vi "get list with seq.vi"(9 "charge state":string, 10 "wheelnumber":string, 11 "runletter":string) -> (3 "Array":string[][](array[string]))   [LabVIEW 2016]
uses:
  <vilib>/addons/database/Connection.llb/DB Tools Open Connec (String).vi
  <vilib>/addons/database/Connection.llb/Conn Execute.vi
  <vilib>/addons/database/Recordset.llb/Rec Fetch Recordset Data (R).vi
  <vilib>/addons/database/Recordset.llb/Rec Destroy - Connection.vi
  <vilib>/addons/database/NI_Database_API.lvlib
  <vilib>/Analysis/NI_AALBase.lvlib
panel:
  out "error out":errorcluster
  out "recordset data":variant[][](array[variant])
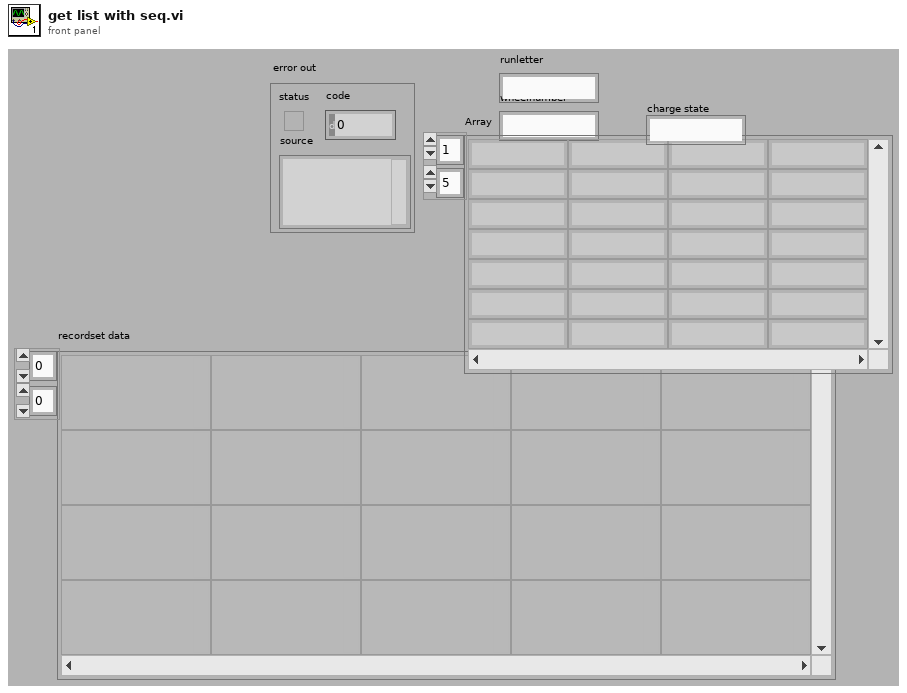
[diagram p1: front panel]
types:
  T1 = typedef "NI_Database_API.lvlib/Conn ObjectReference.ctl" = refnum<k1>
  T2 = typedef "NI_Database_API.lvlib/Rec ObjectReference.ctl" = refnum<k1>
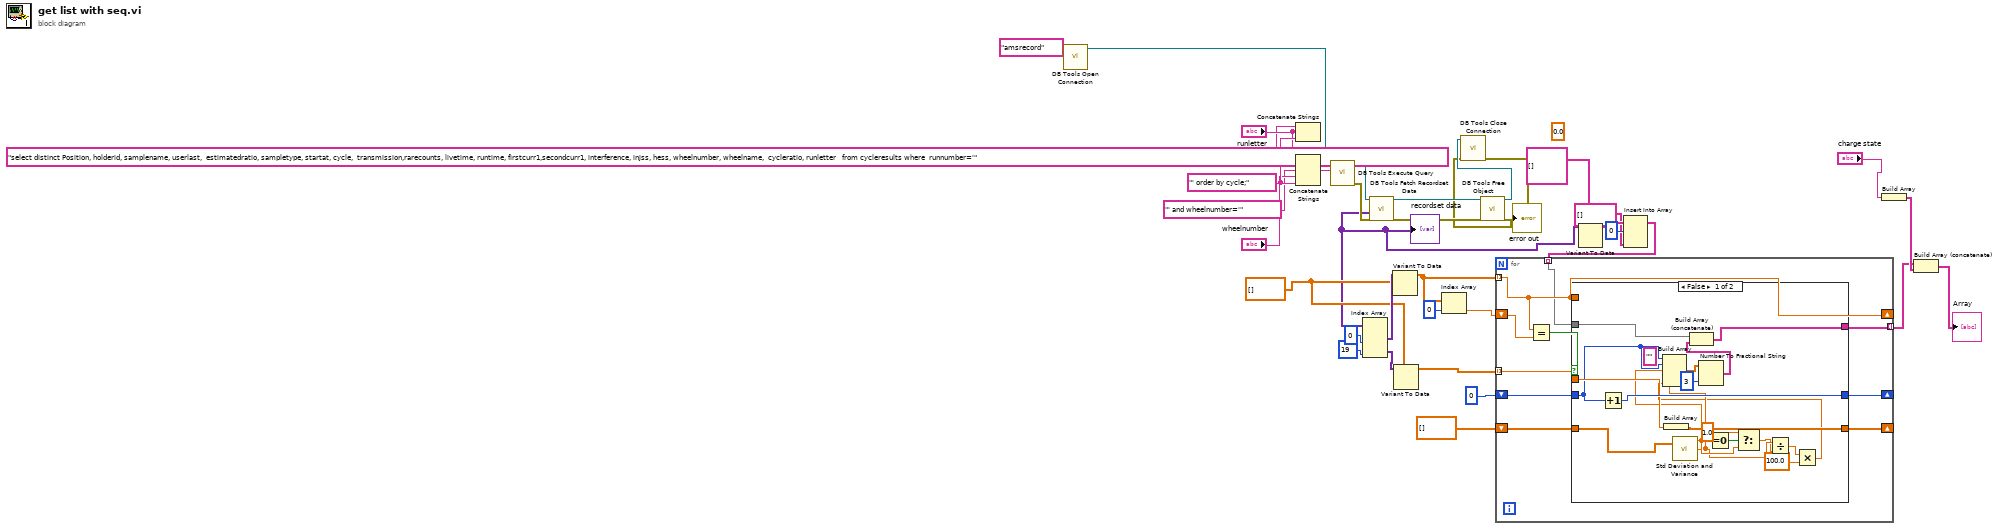
[diagram p0: block diagram]
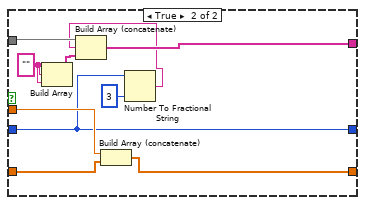
[diagram p2: hidden frame]
diagram:
  (unwired) 0.0
  w21 = dbl[] []
  w34 = "' order by cycle;" ("SQL query get data name")
  w32 = "select distinct Position, holderid, samplename, userlast,  estimatedratio, sampletype, startat, cycle,  transmission,rarecounts, livetime, runtime, firstcurr1,secondcurr1, interference, injss, hess, wheelnumber, wheelname,  cycleratio, runletter   from cycleresults where  runnumber='" ("SQL query get data name")
  n1 = call-poly <vilib>:"DB Tools Open Connection.vi"("connection information"="amsrecord") -> ("connection reference"=w27:T1)  [unwired: 7 in, 1 out]
  n2 = Concatenate Strings(w32, "runletter", w34) -> ()  [unwired: 1 out]
  n3 = Concatenate Strings(w32, "runletter", "' and wheelnumber='" ("SQL query get data name"), "wheelnumber", w34) -> (w35:string)
  n4 = call-poly <vilib>:"DB Tools Execute Query.vi"("SQL query"=w35, "connection reference"=w27) -> ("error out"=w28:errorcluster, "recordset reference"=w29:T2)  [unwired: 6 in]
  n5 = call-poly <vilib>:"DB Tools Fetch Recordset Data.vi"("error in (no error)"=w28, "recordset reference"=w29) -> ("error out"=w25:errorcluster, "recordset data"=w13:variant[][], "recordset reference out"=w26:T2)  [unwired: 3 in]
  "recordset data" <- w13
  n6 = Index Array(array=w13, index (col) #1=0 ("index (row)"), index (col) #2=19 ("disabled index (col)")) -> (element #1=w22:variant[], element #2=w20:variant[])  [unwired: 2 in]
  n7 = Variant To Data(type=w21, Variant=w22) -> (data=w17:dbl[])  [unwired: 1 in, 1 out]
  n8 = Variant To Data(type=w21, Variant=w20) -> (data=w19:dbl[])  [unwired: 1 in, 1 out]
  n9 = Index Array(array=w17, index=0) -> (element=w15:dbl)
  n10 = call-poly <vilib>:"DB Tools Free Object.vi"("error in (no error)"=w25, "recordset reference"=w26) -> ("error out"=w1:errorcluster, "connection reference"=w3:T1)  [unwired: 8 in]
  n11 = call <vilib>:"DB Tools Close Connection.vi"("error in (no error)"=w1, "connection reference"=w3) -> ("error out"=→"error out":errorcluster)  [unwired: 5 in]
  n12 = Variant To Data(type=string[][] [], Variant=w13) -> (data=w11:string[][])  [unwired: 1 in, 1 out]
  n13 = Insert Into Array(array=w11, index (row)=0, new element=string[] [] ("new element/subarray")) -> (w8:string[][])  [unwired: 1 in]
  n14 = for {
    tunnel: w19 -> [w42] mode=indexing
    tunnel: w17 -> [w44] mode=indexing
    shift-right: [w39] -> _
    shift-left: 0 ("index (row)") -> [w46]
    shift-right: [w44] -> _
    shift-left: w15 -> [w45]
    shift-right: [w40] -> _
    shift-left: dbl[] [] -> [w41]
    tunnel: w8 -> [w38] mode=indexing
    tunnel: [w37] -> w5 mode=indexing
    n15 = Equal?(x=w44, y=w45) -> (x = y?=w43:bool)
    n16 = case shown="False" w43 {
      tunnel: w44 -> [_ _]
      tunnel: w46 -> [w56 w68]
      tunnel: w42 -> [w58 w74]
      tunnel: w41 -> [w55 w73]
      tunnel: [w57 w72] -> w40
      tunnel: [w63 w68] -> w39
      tunnel: w38 -> [w64 w71]
      tunnel: [w62 w70] -> w37
      frame False {
        (unwired) ""
        n17 = Increment(x=w56) -> (x+1=w63:i32)
        n18 = Build Array(w58) -> (w57:dbl[])
        n19 = call <vilib>:"Std Deviation and Variance.vi"("X"=w55) -> ("mean"=w53:dbl, "standard deviation"=w51:dbl)  [unwired: 1 in, 1 out]
        n20 = Equal To 0?(x=w53) -> (x = 0?=w54:bool)
        n21 = Select(t=1.0, s=w54, f=w53) -> (s? t:f=w50:dbl)
        n22 = Divide(x=w51, y=w50) -> (x/y=w49:dbl)
        n23 = Multiply(x=w49, y=100.0) -> (x*y=w47:dbl)
        n24 = Build Array(w56, w56, w53, w51, w47) -> (w61:dbl[])
        n25 = Number To Fractional String(number=w61, precision (6)=i16 3) -> (F-format string=w60:string[])  [unwired: 2 in]
        n26 = Build Array (concatenate)(w64, w60) -> (w62:string[])
      }
      frame True {
        w65 = ""
        n27 = Build Array(w65, w65, w65) -> (w67:string[])
        n28 = Build Array (concatenate)(w74, w73) -> (w72:dbl[])
        n29 = Number To Fractional String(number=w68, precision (6)=i16 3) -> (F-format string=w66:string)  [unwired: 2 in]
        n30 = Build Array (concatenate)(w71, w66, w67) -> (w70:string[])
      }
    }
  }
  n31 = Build Array("charge state") -> (w6:string[])
  n32 = Build Array (concatenate)(w5, w6) -> (→"Array":string[][])
